vi "mlProject_testHoloNet.vi"() -> ()   [LabVIEW 2016]
uses:
  <vilib>/Analysis/2dsp.llb/2D Real FFT.vi
  <vilib>/Analysis/NI_AALPro.lvlib
panel:
  out "Runs":i32
  out "Error":sgl[](graph)
  in  "forward?":bool
  in  "eta":sgl
  out "Intensity Graph":sgl[][](graph)
  out "Intensity Graph 2":dbl[][](graph)
  out "address":i64
  in  "milliseconds to wait":u32
  in  "stop":bool
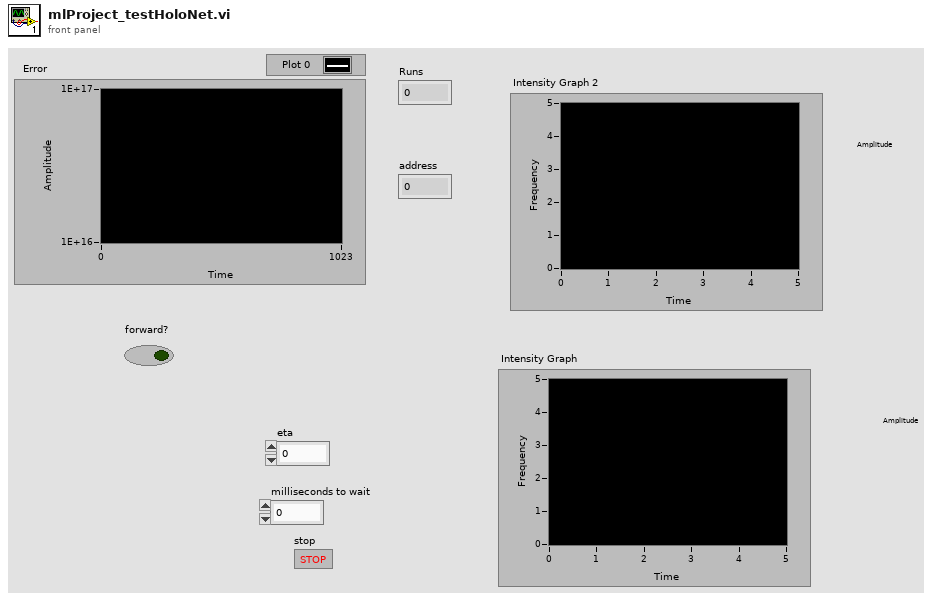
[diagram p1: front panel]
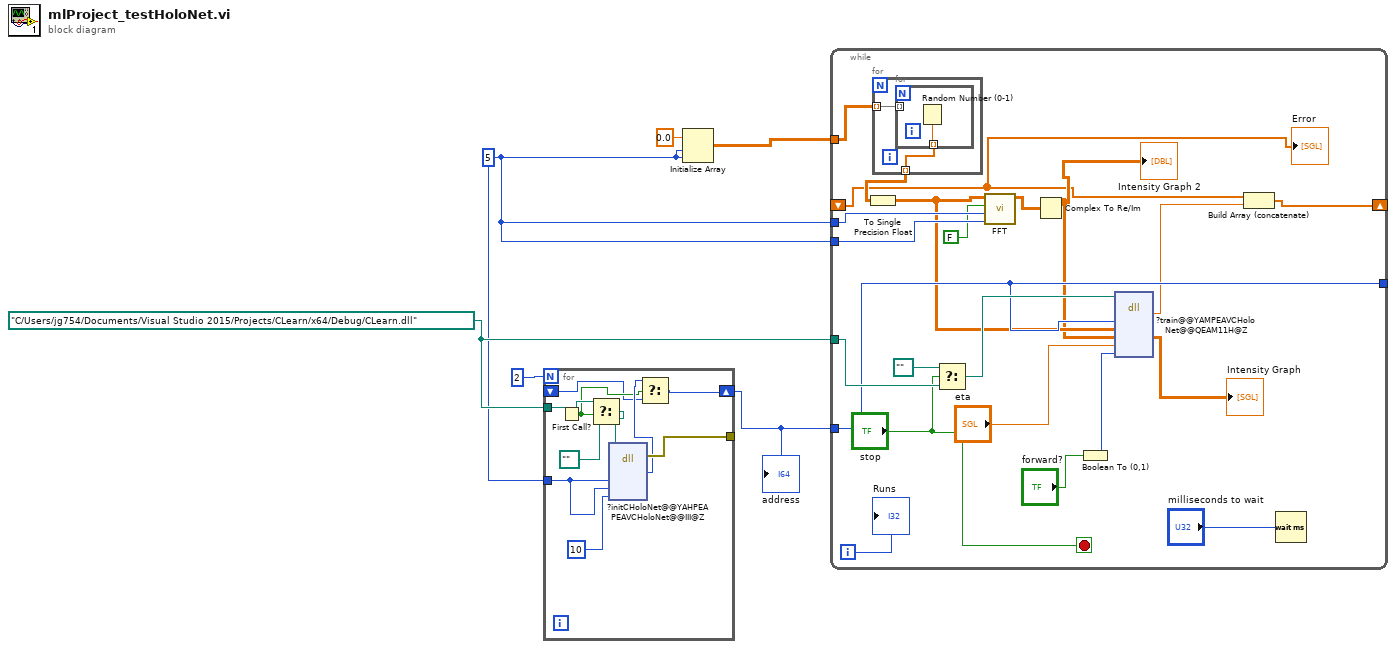
[diagram p0: block diagram]
diagram:
  w1 = u32 5 ("dimension size")
  w4 = path "C:/Users/jg754/Documents/Visual Studio 2015/Projects/CLearn/x64/Debug/CLearn.dll" ("path in")
  n1 = for {
    N: 2 -> [_]
    tunnel: w4 -> [w15]
    tunnel: [w16] -> _
    shift-right: [w12] -> w5
    shift-left: _ -> [w10]
    tunnel: w1 -> [w8]
    n2 = First Call?() -> (First Call?: T/F=w11:bool)
    n3 = Select(t=w15, s=w11, f=path "") -> (s? t:f=w14:path)
    n4 = dll-call lib="C:/Users/jg754/Documents/Visual Studio 2015/Projects/CLearn/x64/Debug/CLearn.dll" fn="?initCHoloNet@@YAHPEAPEAVCHoloNet@@III@Z"(path in=w14, "NINXY"=w8, "NOUTXY"=w8, "NNODES"=u32 10) -> (error out=w16:errorcluster, "ptr"=w13:i64)  [unwired: 7 in, 1 out]
    n5 = Select(t=w13, s=w11, f=w10) -> (s? t:f=w12:i64)
  }
  "address" <- w5
  n6 = Initialize Array(0.0 ("element"), w1, w1) -> (w2:dbl[][])
  n7 = while {
    tunnel: w5 -> [w28]
    tunnel: w4 -> [w37]
    tunnel: [w28] -> _
    tunnel: w2 -> [w34]
    tunnel: w1 -> [w31]
    tunnel: w1 -> [w30]
    shift-right: [w19] -> _
    shift-left: _ -> [w18]
    i -> [w17]
    stop <- "stop" stop-if-true
    n8 = for {
      tunnel: w34 -> [w40] mode=indexing
      tunnel: [w39] -> w32 mode=indexing
      n9 = for {
        tunnel: w40 -> [_] mode=indexing
        tunnel: [w41] -> w39 mode=indexing
        n10 = Random Number (0-1)() -> (number: 0 to 1=w41:dbl)
      }
    }
    n11 = To Single Precision Float(number=w32) -> (single precision float=w27:sgl[][])
    n12 = Select(t=path "", s="stop", f=w37) -> (s? t:f=w36:path)
    n13 = call-poly <vilib>:"FFT.vi"("n"=w30, "m"=w31, "shift?"=FALSE, "X"=w27) -> ("FFT {X}"=w26:cdb[][])  [unwired: 6 in, 1 out]
    n14 = Complex To Re/Im(x + iy=w26) -> (x=w25:dbl[][])  [unwired: 1 out]
    "Intensity Graph 2" <- w25
    n15 = Boolean To (0,1)(Boolean="forward?") -> (0, 1=w21:i16)
    n16 = dll-call lib="C:/Users/jg754/Documents/Visual Studio 2015/Projects/CLearn/x64/Debug/CLearn.dll" fn="?train@@YAMPEAVCHoloNet@@QEAM11H@Z"(path in=w36, "ptr"=w28, "in"=w27, "dOut"=w25, "eta"="eta", "forwardOnly"=w21) -> ("error"=w20:sgl, "dOut"=→"Intensity Graph":sgl[][])  [unwired: 6 in, 2 out]
    n17 = Build Array (concatenate)(w18, w20) -> (w19:sgl[])
    n18 = Wait (ms)(milliseconds to wait="milliseconds to wait") -> ()  [unwired: 1 out]
    "Error" <- w18
    "Runs" <- w17
  }
